vi "Teleop.vi"(10 "Match Info":T1={"Autonomous Elapsed Seconds"=0.0, "TeleOp Elapsed Seconds"=0.0, "Disabled Elapsed Seconds"=0.0, "Visited Autonomous"=FALSE, "Visited TeleOp"=FALSE, "Visited Disabled"=FALSE, "Autonomous Settings"={"Autonomous Style"=enum."Independent", "VI Refnum"=refnum}}, 11 "Call Context":T2) -> ()   [LabVIEW 2011]
doc: "This VI is called for each TeleOp packet received from the DS where the robot is not disabled. It is often used to read from the joysticks and update I/O or to update setpoints for timed control loops. It should complete and return within 20 milliseconds or it may miss DS packets."
uses:
  <vilib>/Rock Robotics/WPI/DriverStation/WPI_DriverStationDerivedRobotMode.ctl
  <vilib>/Rock Robotics/WPI/DriverStation/WPI_DriverStationMatch Info.ctl
  <vilib>/Rock Robotics/WPI/Joystick/WPI_JoystickAxis.ctl
  <vilib>/Rock Robotics/WPI/Solenoid/WPI_SolenoidValue.ctl
  Robot Global Data.vi
  <vilib>/Rock Robotics/WPI/Solenoid/WPI_SolenoidGetEnum.vi
  <vilib>/Rock Robotics/WPI/Solenoid/WPI_SolenoidSetEnum.vi
panel:
  in  "upper limit":dbl=1.0
  in  "Key Speed":dbl=0.85
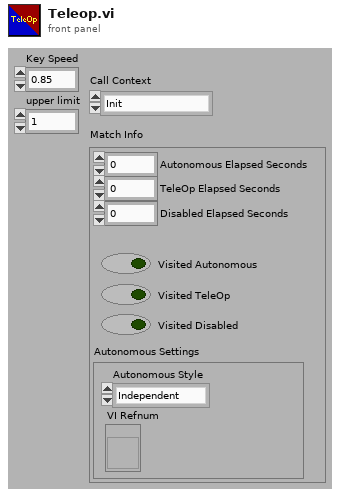
[diagram p1: front panel]
types:
  T1 = typedef "WPI_DriverStationMatch Info.ctl" = cluster{"Autonomous Elapsed Seconds":dbl, "TeleOp Elapsed Seconds":dbl, "Disabled Elapsed Seconds":dbl, "Visited Autonomous":bool, "Visited TeleOp":bool, "Visited Disabled":bool, "Autonomous Settings":cluster{"Autonomous Style":enum16{"Iterative", "Independent"}, "VI Refnum":refnum<vi>}}
  T2 = typedef "WPI_DriverStationDerivedRobotMode.ctl" = enum16{"Init", "Execute", "Stop"}
  T3 = typedef "WPI_JoystickAxis.ctl" = enum16{"Axis 1", "Axis 2", "Axis 3", "Axis 4", "Axis 5", "Axis 6"}
  T4 = typedef "WPI_SolenoidValue.ctl" = enum16{"Off", "On", "Forward", "Reverse"}
  T5 = typedef "WPI_JoystickDevRef.ctl" = cluster{"Device":T6}
  T6 = typedef "WPI_JoystickDeviceEnum.ctl" = enum16{"USB 1", "USB 2", "USB 3", "USB 4", "Kinect 1", "Kinect 2"}
  T7 = typedef "WPI_JoystickButtonState.ctl" = cluster{"Button 1":bool, "Button 2":bool, "Button 3":bool, "Button 4":bool, "Button 5":bool, "Button 6":bool, "Button 7":bool, "Button 8":bool, "Button 9":bool, "Button 10":bool, "Button 11":bool, "Button 12":bool}
  T8 = typedef "WPI_RobotDriveDevRef.ctl" = cluster{"DevStatus":errorcluster, "Motors[]":T9[], "Square Inputs":bool, "Max Output":dbl, "Isochronous":bool}
  T9 = typedef "WPI_MotorControlDeviceRef.ctl" = cluster{"DeviceStatus":errorcluster, "Type":enum16{"PWM", "CAN"}, "PWM":cluster{"Digital Module":T10, "PWM Channel":T11, "DeadBand":T12}, "CAN":cluster{"Device Number":u8, "Control Mode":T13, "Semaphore":T14, "Max Vout":dbl}, "Invert":bool, "TransformRef":T15, "InvTransformRef":T15}
  T10 = typedef "FPGA_TypedefDigitalModule.ctl" = enum16{"Digital Module 1", "Digital Module 2"}
  T11 = typedef "FPGA_DIOPWMChannel.ctl" = enum8{"PWM 1", "PWM 2", "PWM 3", "PWM 4", "PWM 5", "PWM 6", "PWM 7", "PWM 8", "PWM 9", "PWM 10", "Invalid"}
  T12 = typedef "WPI_PWMDeadband.ctl" = cluster{"Name":string, "maxPositivePwm":i32, "minPositivePwm":i32, "centerPwm":i32, "maxNegativePwm":i32, "minNegativePwm":i32, "angularRange":u16}
  T13 = typedef "WPI_CANJaguar_ControlMode.ctl" = enum8{"Percent VBus", "Current", "Speed", "Position", "Voltage"}
  T14 = typedef "Semaphore RefNum" = refnum<k1>
  T15 = typedef "WPI_PWMTransform_ConPane.ctl" = refnum<vi>
  T16 = typedef "WPI_SolenoidDevRef.ctl" = cluster{"DevStatus":errorcluster, "Solenoid Module":T17, "Forward Solenoid Channel":T18, "Reverse Solenoid Channel":T18}
  T17 = typedef "FPGA_TypedefSolenoidModule.ctl" = enum16{"Solenoid Module 1", "Solenoid Module 2"}
  T18 = typedef "WPI_SolenoidChannel.ctl" = enum8{"Solenoid 1", "Solenoid 2", "Solenoid 3", "Solenoid 4", "Solenoid 5", "Solenoid 6", "Solenoid 7", "Solenoid 8", "Invalid"}
  T19 = typedef "WPI_ServoDeviceRef.ctl" = cluster{"DeviceStatus":errorcluster, "Digital Module":T10, "PWM Channel":T11, "DeadBand":T12}
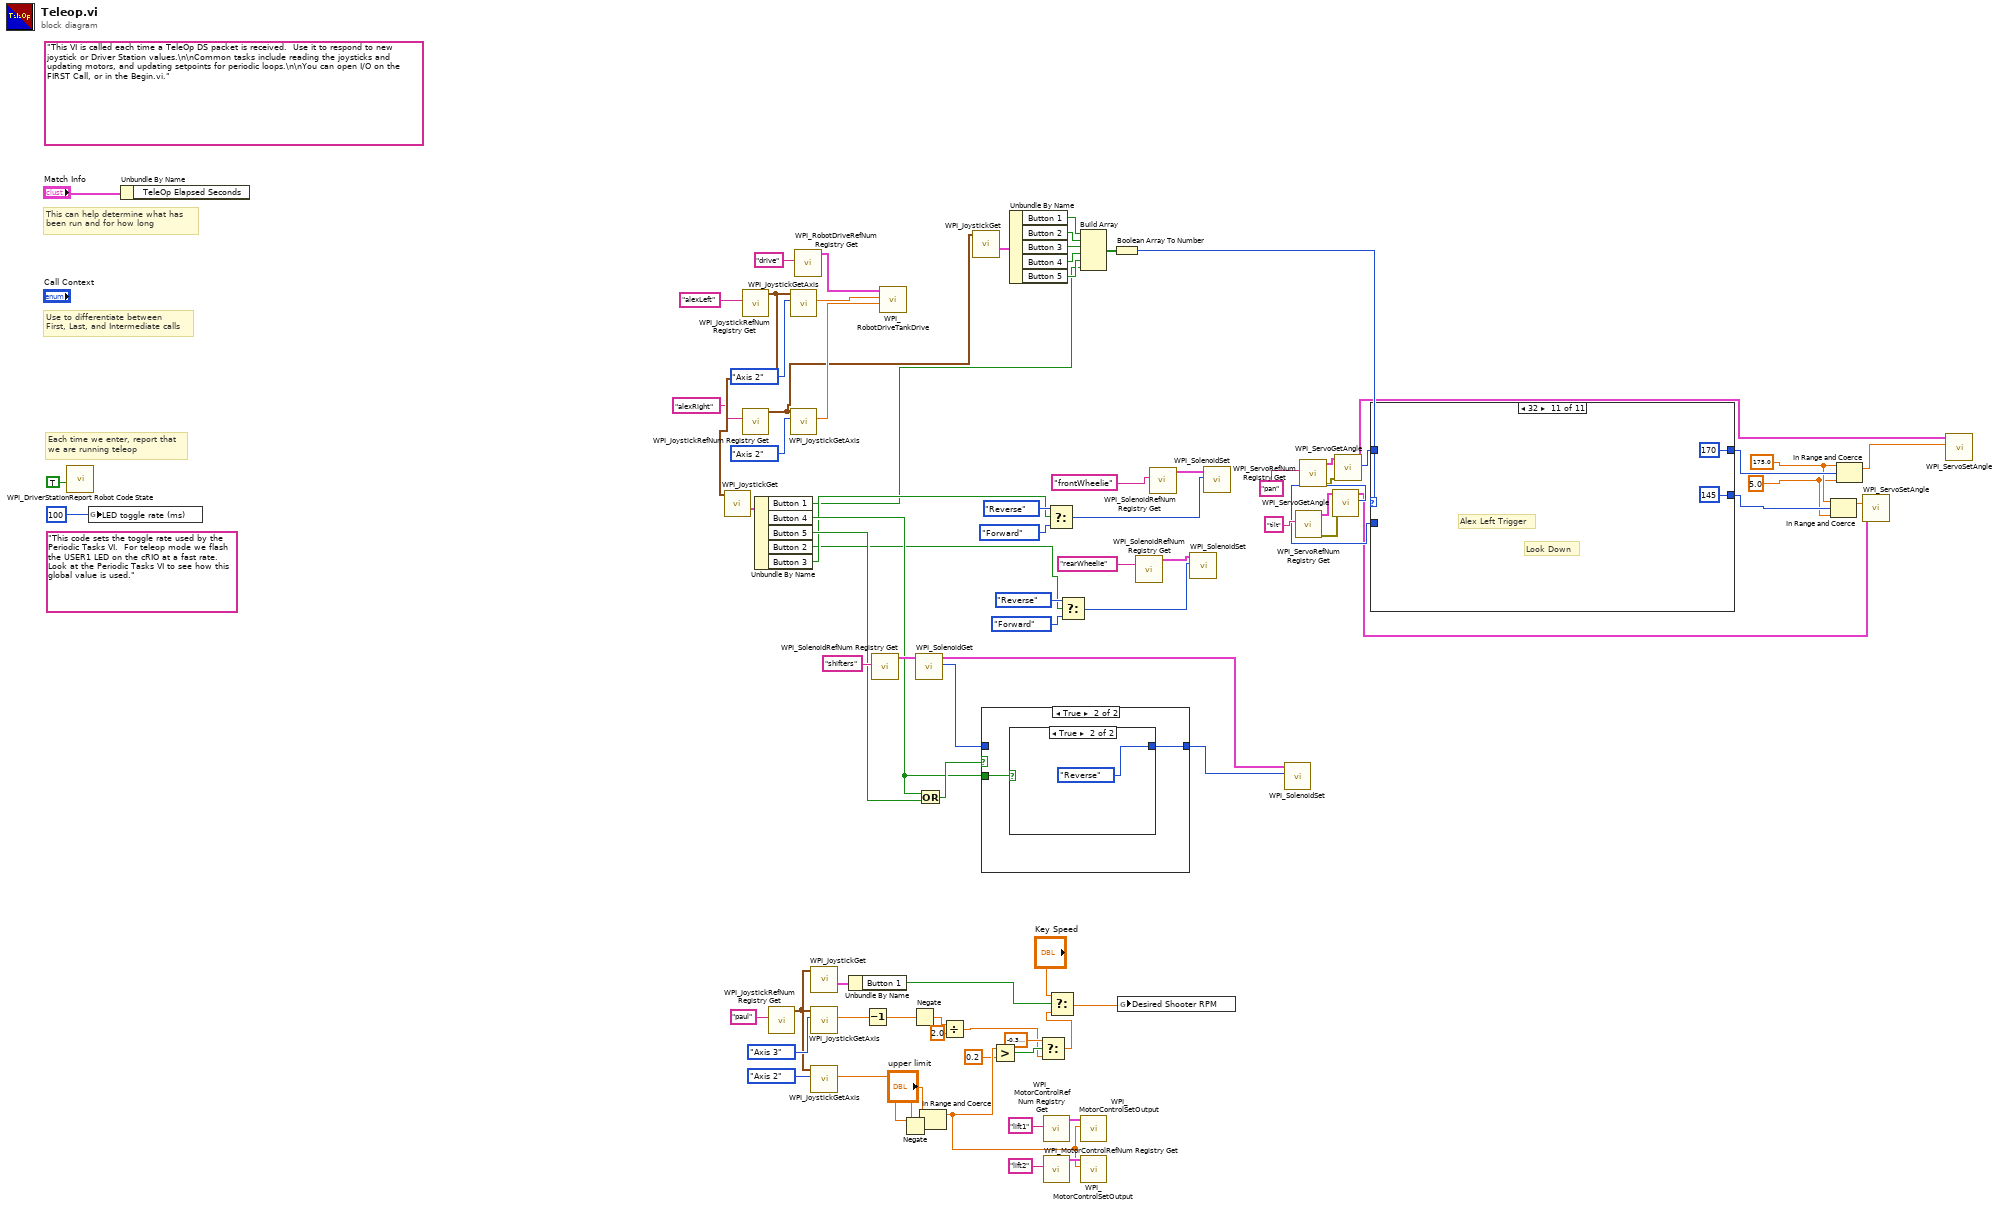
[diagram p0: block diagram]
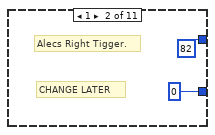
[diagram p3: hidden frame]
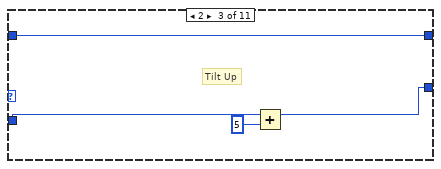
[diagram p4: hidden frame]
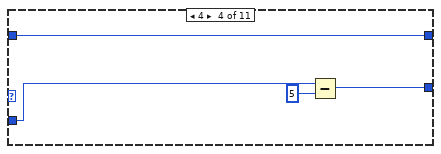
[diagram p5: hidden frame]
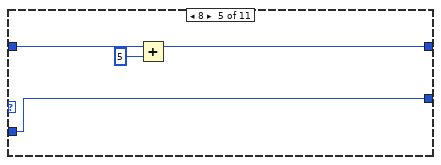
[diagram p6: hidden frame]
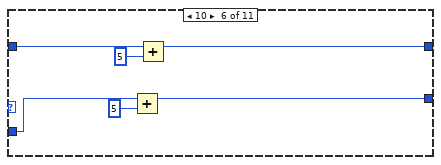
[diagram p7: hidden frame]
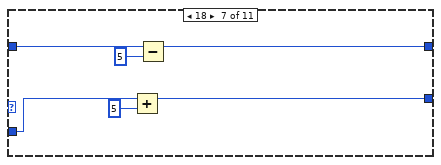
[diagram p8: hidden frame]
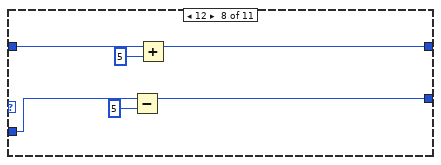
[diagram p9: hidden frame]
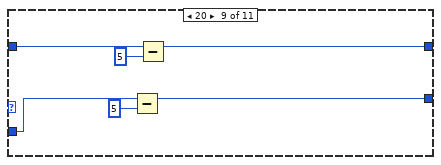
[diagram p10: hidden frame]
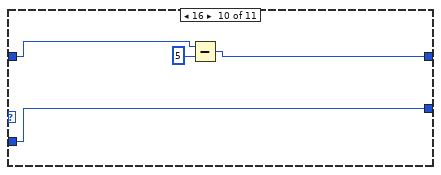
[diagram p11: hidden frame]
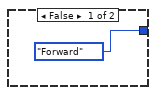
[diagram p13: hidden frame]
diagram:
  w11 = 5.0 ("lower limit")
  w12 = 175.0 ("upper limit")
  (unwired) "This code sets the toggle rate used by the Periodic Tasks VI.  For teleop mode we flash the USER1 LED on the cRIO at a fast rate.  Look at the Periodic Tasks VI to see how this global value is used."
  (unwired) "This VI is called each time a TeleOp DS packet is received.  Use it to respond to new joystick or Driver Station values.\n\nCommon tasks include reading the joysticks and updating motors, and updating setpoints for periodic loops.\n\nYou can open I/O on the FIRST Call, or in the Begin.vi."
  # "Each time we enter, report that\nwe are running teleop"
  # "Use to differentiate between\nFirst, Last, and Intermediate calls"
  # "This can help determine what has\nbeen run and for how long"
  n1 = call <vilib>:"WPI_DriverStationReport Robot Code State.vi"("TeleOp"=TRUE ("Autonomous")) -> ()  [unwired: 10 in, 1 out]
  n2 = global write "Robot Global Data.vi" "LED toggle rate (ms)"(u32 100 ("LED ms toggle rate")) -> ()
  n3 = Unbundle By Name("Match Info") -> ()  [unwired: 1 out]
  n4 = call <vilib>:"WPI_JoystickRefNum Registry Get.vi"("refnum name"="alexLeft") -> ("JoystickDevRef"=w44:T5)  [unwired: 9 in, 1 out]
  n5 = call <vilib>:"WPI_JoystickGet.vi"("JoystickDevRef"=w44) -> ("Buttons"=w65:T7)  [unwired: 4 in, 2 out]
  n6 = call <vilib>:"WPI_JoystickRefNum Registry Get.vi"("refnum name"="alexRight") -> ("JoystickDevRef"=w41:T5)  [unwired: 9 in, 1 out]
  n7 = Unbundle By Name(w65) -> ("Button 1"=w29:bool, "Button 4"=w37:bool, "Button 5"=w38:bool, "Button 2"=w35:bool, "Button 3"=w36:bool)
  n8 = call <vilib>:"WPI_JoystickRefNum Registry Get.vi"("refnum name"="paul") -> ("JoystickDevRef"=w48:T5)  [unwired: 9 in, 1 out]
  n9 = call <vilib>:"WPI_JoystickGetAxis.vi"("Axis"=WPI_JoystickAxis."Axis 2", "JoystickDevRef"=w44) -> ("Value"=w80:dbl)  [unwired: 8 in, 1 out]
  n10 = call <vilib>:"WPI_JoystickGetAxis.vi"("Axis"=WPI_JoystickAxis."Axis 2", "JoystickDevRef"=w41) -> ("Value"=w81:dbl)  [unwired: 8 in, 1 out]
  n11 = call <vilib>:"WPI_RobotDriveRefNum Registry Get.vi"("refnum name"="drive") -> ("RobotDriveDevRef"=w76:T8)  [unwired: 1 in, 9 out]
  n12 = call <vilib>:"WPI_JoystickGet.vi"("JoystickDevRef"=w48) -> ("Buttons"=w47:T7)  [unwired: 4 in, 2 out]
  n13 = call <vilib>:"WPI_JoystickGetAxis.vi"("Axis"=WPI_JoystickAxis."Axis 3", "JoystickDevRef"=w48) -> ("Value"=w45:dbl)  [unwired: 8 in, 1 out]
  n14 = call <vilib>:"WPI_JoystickGetAxis.vi"("Axis"=WPI_JoystickAxis."Axis 2", "JoystickDevRef"=w48) -> ("Value"=w10:dbl)  [unwired: 8 in, 1 out]
  n15 = Unbundle By Name(w47) -> ("Button 1"=w46:bool)
  n16 = Decrement(x=w45) -> (x-1=w50:dbl)
  n17 = call <vilib>:"WPI_SolenoidRefNum Registry Get.vi"("refnum name"="shifters") -> ("SolenoidDevRef"=w61:T16)  [unwired: 9 in, 1 out]
  n18 = call <vilib>:"WPI_RobotDriveTankDrive.vi"("Right axis value"=w81, "Left axis value"=w80, "RobotDriveDevRef"=w76) -> ()  [unwired: 7 in, 2 out]
  n19 = Negate(x="upper limit") -> (-x=w8:dbl)
  n20 = Negate(x=w50) -> (-x=w40:dbl)
  n21 = call-poly <vilib>:"WPI_SolenoidGet.vi"("SolenoidDevRef"=w61) -> ("Value"=w59:T4, "SolenoidDevRef"=w60:T16)  [unwired: 8 in, 1 out]
  n22 = Or(x=w37, y=w38) -> (x .or. y?=w62:bool)
  n23 = In Range and Coerce(upper limit="upper limit", x=w10, lower limit=w8) -> (coerced(x)=w7:dbl)  [unwired: 1 out]
  n24 = Divide(x=w40, y=2.0) -> (x/y=w1:dbl)
  n25 = call <vilib>:"WPI_JoystickGet.vi"("JoystickDevRef"=w41) -> ("Buttons"=w43:T7)  [unwired: 4 in, 2 out]
  n26 = case shown="True" w62 {
    tunnel: w59 -> [w85 _]
    tunnel: [w85 w87] -> w58
    tunnel: w37 -> [_ w86]
    frame False {
    }
    frame True {
      n27 = case shown="True" w86 {
        tunnel: [WPI_SolenoidValue."Forward" ("Value") WPI_SolenoidValue."Reverse" ("Value")] -> w87
        frame False {
        }
        frame True {
        }
      }
    }
  }
  n28 = Greater?(x=w7, y=0.2) -> (0:w5:bool)
  n29 = Unbundle By Name(w43) -> ("Button 1"=w34:bool, "Button 2"=w33:bool, "Button 3"=w32:bool, "Button 4"=w31:bool, "Button 5"=w30:bool)
  n30 = Select(t=-0.39999999999999997, s=w5, f=w1) -> (s? t:f=w2:dbl)
  n31 = call <vilib>:"WPI_MotorControlRefNum Registry Get.vi"("refnum name"="lift1") -> ("MotorControlDevRef"=w54:T9)  [unwired: 9 in, 1 out]
  n32 = call <vilib>:"WPI_MotorControlRefNum Registry Get.vi"("refnum name"="lift2") -> ("MotorControlDevRef"=w53:T9)  [unwired: 9 in, 1 out]
  n33 = Select(t=WPI_SolenoidValue."Reverse" ("Value"), s=w36, f=WPI_SolenoidValue."Forward" ("Value")) -> (s? t:f=w64:T4)
  n34 = Select(t="Key Speed", s=w46, f=w2) -> (s? t:f=w3:dbl)
  n35 = Select(t=WPI_SolenoidValue."Reverse" ("Value"), s=w35, f=WPI_SolenoidValue."Forward" ("Value")) -> (s? t:f=w63:T4)
  n36 = Build Array(w34, w33, w32, w31, w30, w29) -> (w28:bool[])
  n37 = call <vilib>:"WPI_MotorControlSetOutput.vi"("Output"=w7, "MotorControlDevRef"=w54) -> ()  [unwired: 8 in, 2 out]
  n38 = call <vilib>:"WPI_MotorControlSetOutput.vi"("Output"=w7, "MotorControlDevRef"=w53) -> ()  [unwired: 8 in, 2 out]
  n39 = Boolean Array To Number(Boolean array=w28) -> (number=w27:u32)
  n40 = global write "Robot Global Data.vi" "Desired Shooter RPM"(w3) -> ()
  n41 = call <vilib>:"WPI_SolenoidRefNum Registry Get.vi"("refnum name"="rearWheelie") -> ("SolenoidDevRef"=w71:T16)  [unwired: 9 in, 1 out]
  n42 = call <vilib>:"WPI_SolenoidRefNum Registry Get.vi"("refnum name"="frontWheelie") -> ("SolenoidDevRef"=w70:T16)  [unwired: 9 in, 1 out]
  n43 = call-poly <vilib>:"WPI_SolenoidSet.vi"("Value"=w63, "SolenoidDevRef"=w71) -> ()  [unwired: 8 in, 2 out]
  n44 = call-poly <vilib>:"WPI_SolenoidSet.vi"("Value"=w64, "SolenoidDevRef"=w70) -> ()  [unwired: 8 in, 2 out]
  n45 = call-poly <vilib>:"WPI_SolenoidSet.vi"("Value"=w58, "SolenoidDevRef"=w60) -> ()  [unwired: 8 in, 2 out]
  n46 = call <vilib>:"WPI_ServoRefNum Registry Get.vi"("refnum name"="tilt") -> ("error out"=w24:errorcluster, "ServoDeviceRef"=w25:T19)  [unwired: 9 in]
  n47 = call <vilib>:"WPI_ServoRefNum Registry Get.vi"("refnum name"="pan") -> ("error out"=w21:errorcluster, "ServoDeviceRef"=w22:T19)  [unwired: 9 in]
  n48 = call <vilib>:"WPI_ServoGetAngle.vi"("ServoDeviceRef"=w25, "error in (no error)"=w24) -> ("ServoDeviceRef"=w18:T19, "Angle"=w23:u16)  [unwired: 6 in, 1 out]
  n49 = call <vilib>:"WPI_ServoGetAngle.vi"("ServoDeviceRef"=w22, "error in (no error)"=w21) -> ("ServoDeviceRef"=w19:T19, "Angle"=w20:u16)  [unwired: 6 in, 1 out]
  n50 = case shown="32" w27 {
    tunnel: w23 -> [w91 _ w96 w100 w105 w111 w117 w123 w129 w133 _]
    tunnel: [w91 u16 0 ("Angle") w95 w99 w105 w107 w113 w119 w125 w133 u16 145 ("Angle")] -> w13
    tunnel: w20 -> [w90 _ w97 w101 w104 w110 w116 w122 w128 w131 _]
    tunnel: [w90 u16 82 ("Angle") w97 w101 w103 w109 w115 w121 w127 w132 u16 170 ("Angle")] -> w16
    frame 0, Default {
    }
    frame 1 {
      # "Alecs Right Tigger."
      # "CHANGE LATER"
    }
    frame 2 {
      # "Tilt Up"
      n51 = Add(x=w96, y=u16 5) -> (x+y=w95:u16)
    }
    frame 4 {
      n52 = Subtract(x=w100, y=u16 5) -> (x-y=w99:u16)
    }
    frame 8 {
      n53 = Add(x=w104, y=u16 5) -> (x+y=w103:u16)
    }
    frame 10 {
      n54 = Add(x=w111, y=u16 5) -> (x+y=w107:u16)
      n55 = Add(x=w110, y=u16 5) -> (x+y=w109:u16)
    }
    frame 18 {
      n56 = Add(x=w117, y=u16 5) -> (x+y=w113:u16)
      n57 = Subtract(x=w116, y=u16 5) -> (x-y=w115:u16)
    }
    frame 12 {
      n58 = Subtract(x=w123, y=u16 5) -> (x-y=w119:u16)
      n59 = Add(x=w122, y=u16 5) -> (x+y=w121:u16)
    }
    frame 20 {
      n60 = Subtract(x=w129, y=u16 5) -> (x-y=w125:u16)
      n61 = Subtract(x=w128, y=u16 5) -> (x-y=w127:u16)
    }
    frame 16 {
      n62 = Subtract(x=w131, y=u16 5) -> (x-y=w132:u16)
    }
    frame 32 {
      # "Look Down"
      # "Alex Left Trigger"
    }
  }
  n63 = In Range and Coerce(upper limit=w12, x=w13, lower limit=w11) -> (coerced(x)=w14:dbl)  [unwired: 1 out]
  n64 = In Range and Coerce(upper limit=w12, x=w16, lower limit=w11) -> (coerced(x)=w15:dbl)  [unwired: 1 out]
  n65 = call <vilib>:"WPI_ServoSetAngle.vi"("Angle"=w14, "ServoDeviceRef"=w18) -> ()  [unwired: 8 in, 2 out]
  n66 = call <vilib>:"WPI_ServoSetAngle.vi"("Angle"=w15, "ServoDeviceRef"=w19) -> ()  [unwired: 8 in, 2 out]
